vi "GlobalPoseAndTargeting.vi"() -> ()   [LabVIEW 2020]
doc: "This global variable contains sensor readings."
panel:
  out "Apply_Grid_Calibration":bool
  out "Current_Blue_Calibration":dbl
  out "New_Blue_Calibration":dbl
  out "Current_Red_Calibration":dbl
  out "New_Red_Calibration":dbl
  out "Distance_to_Target (in)":dbl
  out "Heading_to_Target (deg)":dbl
  out "Pointed_at_Target":bool
  out "Robot_P (deg)":dbl
  out "CON_Field_Width (in)":dbl
  out "CON_Field_Length (in)":dbl
  out "Robot_Y_Odometry_Only (in)":dbl
  out "Robot_X_Odometry_Only (in)":dbl
  out "Robot_Yaw_Rate (deg/s)":dbl
  out "Vision_Fault":bool
  out "Targeting_Information":dbl[](array[numeric])
  out "Swerve_Ground_Velocity_Heading (deg) [0,360]":dbl
  out "Swerve_Ground_Speed (ft/s)":dbl
  out "Time_Since_Pose_Update (ms)":u32
  out "Set_Robot_Pos":bool
  out "Set_Robot_Y (in)":dbl
  out "Set_Robot_X (in)":dbl
  out "IMU_Failure":bool
  out "Vision_Valid":bool
  out "Robot_H (deg)":dbl
  out "Push_Robot_H (deg)":dbl
  out "Push_Robot_Pos":bool
  out "Push_Robot_Y (in)":dbl
  out "Push_Robot_X (in)":dbl
  out "Robot_Y (in)":dbl
  out "Robot_X (in)":dbl
  # "TARGETING INFORMATION"
  # "CONSTANTS"
  # "ROBOT POSE"
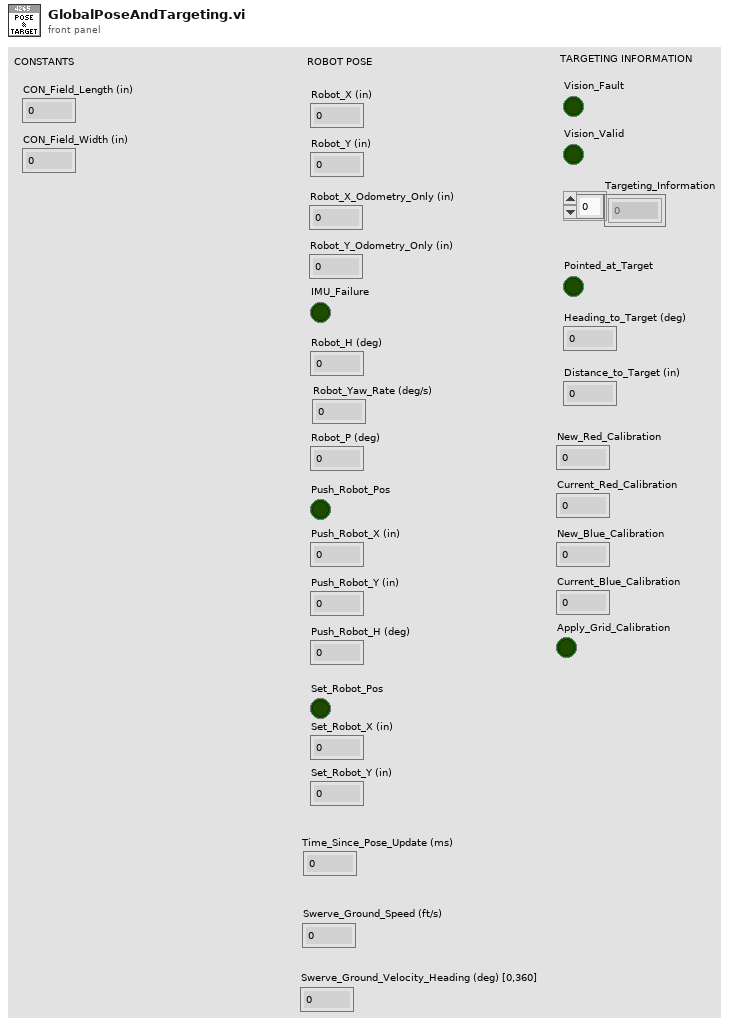
[diagram p1: front panel]
diagram:
